vi "Pump Start Detector (Kuhnke).vi"(6 "Reset":bool, 10 "Window":i32, 11 "Pos Cross":bool) -> (3 "Starts":u32)   [LabVIEW 2019]
uses:
  <vilib>/Platform/TimedLoop/XDataNode/timing_clust.ctl
  <vilib>/Platform/TimedLoop/XDataNode/nitl_modes.ctl
  <vilib>/Platform/TimedLoop/XDataNode/wakeup.ctl
  <vilib>/Platform/TimedLoop/XDataNode/XDataNode.xnode
  <vilib>/Platform/TimedLoop/XDataNode/XDNodeRunTimeDep.lvlib
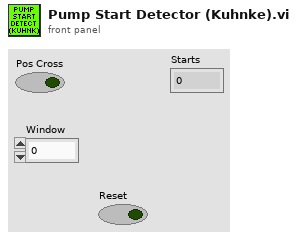
[diagram p1: front panel]
types:
  T1 = typedef "XDNodeRunTimeDep.lvlib/timing_clust.ctl" = cluster{"Expected End [f-1]":u64, "Actual End [f-1]":u64, "Finished Late? [f-1]":bool, "Expected End [i-1]":u64, "Actual End [i-1]":u64, "Finished Late? [i-1]":bool, "Expected Start [i]":u64, "Actual Start [i]":u64, "Expected Start [f]":u64, "Actual Start [f]":u64, "Source Name":string, "Structure Name":string, "Period":i64, "Deadline":i64, "Offset":i64, "Start":i64, "Priority":i32, "Timeout":i32, "Mode":T2, "Wakeup Reason":T3, "Error":errorcluster, "Source Type":string, "Secondary Source Type":string, "Global End Time":u64, "Global Start Time":u64, "Frame Duration":u64, "Iteration Duration":u64, "Assigned CPU":i32, "I/O Scan Engine Mode":u32}
  T2 = typedef "XDNodeRunTimeDep.lvlib/nitl_modes.ctl" = enum32{"No Change", "Process missed periods, maintain original phase", "Discard missed periods, maintain original phase", "Process missed periods, ignore original phase", "Discard missed periods, ignore original phase"}
  T3 = typedef "XDNodeRunTimeDep.lvlib/wakeup.ctl" = enum32{"Normal", "Aborted", "Asynchronous wakeup", "Timing source error", "Timed loop error", "Timeout"}
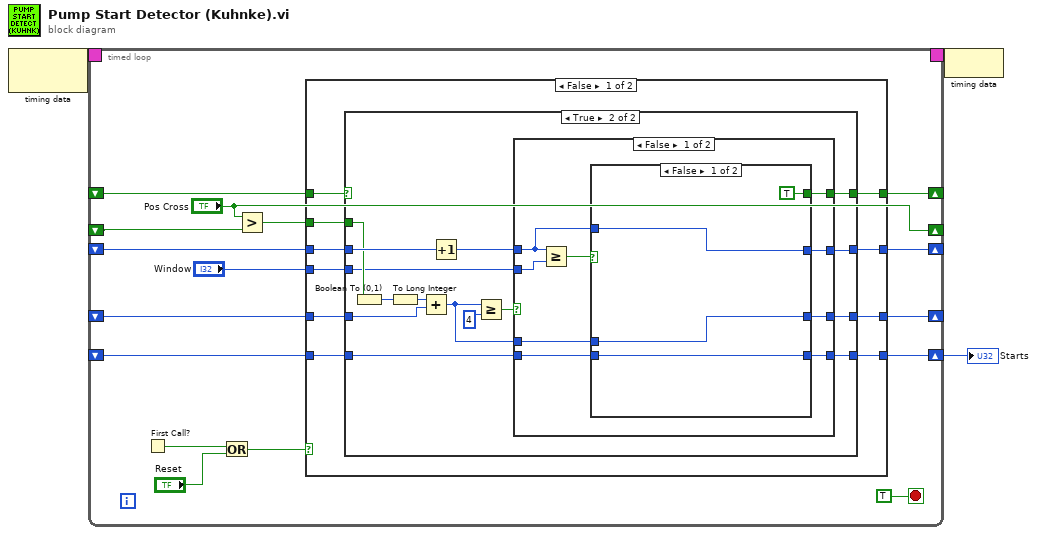
[diagram p0: block diagram]
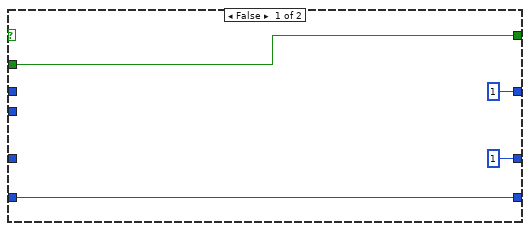
[diagram p2: hidden frame]
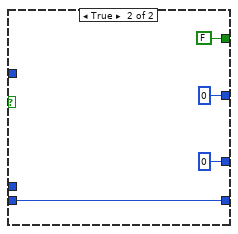
[diagram p3: hidden frame]
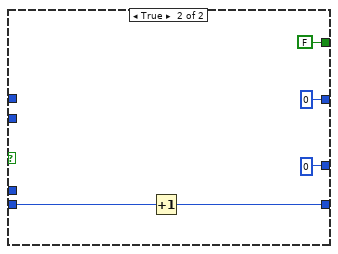
[diagram p4: hidden frame]
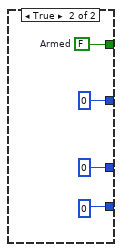
[diagram p5: hidden frame]
diagram:
  n1 = node-c288() -> (w3:T1)  [unwired: 1 in]
  n2 = timed-loop {
    shift-right: [w13] -> w1
    shift-left: _ -> [w14]
    shift-right: [w18] -> _
    shift-left: _ -> [w19]
    shift-right: [w17] -> _
    shift-left: _ -> [w16]
    timing: w3 -> [_]
    timing-out: [_] -> w2
    shift-right: ["Pos Cross"] -> _
    shift-left: _ -> [w9]
    shift-right: [w7] -> _
    shift-left: _ -> [w6]
    stop <- TRUE stop-if-true
    n3 = First Call?() -> (First Call?: T/F=w12:bool)
    n4 = Or(x=w12, y="Reset") -> (x .or. y?=w11:bool)
    n5 = Greater?(x="Pos Cross", y=w9) -> (0:w8:bool)
    n6 = case shown="False" w11 {
      tunnel: w19 -> [w29 _]
      tunnel: [w28 w72] -> w18
      tunnel: [w26 0] -> w17
      tunnel: w16 -> [w24 _]
      tunnel: w14 -> [w22 _]
      tunnel: [w21 u32 0] -> w13
      tunnel: "Window" -> [w20 _]
      tunnel: w8 -> [w27 _]
      tunnel: [w25 0] -> w7
      tunnel: w6 -> [w23 _]
      frame False {
        n7 = case shown="True" w29 {
          tunnel: [w33 w40] -> w28
          tunnel: w27 -> [w33 w47]
          tunnel: [1 ("Window") w39] -> w26
          tunnel: [1 ("Window") w41] -> w25
          tunnel: w24 -> [_ w48]
          tunnel: w23 -> [_ w36]
          tunnel: w22 -> [w30 w43]
          tunnel: [w30 w42] -> w21
          tunnel: w20 -> [_ w37]
          frame False {
          }
          frame True {
            n8 = Boolean To (0,1)(Boolean=w47) -> (0, 1=w46:i16)
            n9 = To Long Integer(number=w46) -> (32bit integer=w34:i32)
            n10 = Add(x=w34, y=w36) -> (x+y=w35:i32)
            n11 = Increment(x=w48) -> (x+1=w38:i32)
            n12 = Greater Or Equal?(x=w35, y=4) -> (x >= y?=w44:bool)
            n13 = case shown="False" w44 {
              tunnel: w43 -> [w55 w70]
              tunnel: [w54 w69] -> w42
              tunnel: [w53 0 ("Window")] -> w41
              tunnel: [w51 FALSE] -> w40
              tunnel: [w52 0 ("Window")] -> w39
              tunnel: w38 -> [w50 _]
              tunnel: w37 -> [w57 _]
              tunnel: w35 -> [w49 _]
              frame False {
                n14 = Greater Or Equal?(x=w50, y=w57) -> (x >= y?=w56:bool)
                n15 = case shown="False" w56 {
                  tunnel: [w61 w65] -> w54
                  tunnel: w55 -> [w61 w65]
                  tunnel: [w58 0 ("Window")] -> w53
                  tunnel: [w60 0 ("Window")] -> w52
                  tunnel: [TRUE FALSE] -> w51
                  tunnel: w50 -> [w60 _]
                  tunnel: w49 -> [w58 _]
                  frame False {
                  }
                  frame True {
                  }
                }
              }
              frame True {
                n16 = Increment(x=w70) -> (x+1=w69:u32)
              }
            }
          }
        }
      }
      frame True {
        w72 = FALSE  # Armed
      }
    }
  }
  "Starts" <- w1
  n17 = node-c288(w2) -> ()
